vi "Encoder SD Write.vi"(9 "Encoder Data":T1 {"Ticks" format="%#.6g"}, 11 "Name":string) -> ()   [LabVIEW 2013]
uses:
  Single Encoder Data.ctl
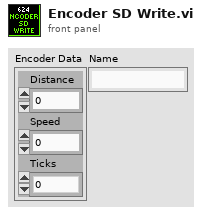
[diagram p1: front panel]
types:
  T1 = typedef "Single Encoder Data.ctl" = cluster{"Distance":dbl, "Speed":dbl, "Ticks":dbl}
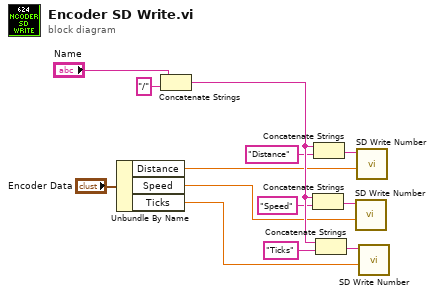
[diagram p0: block diagram]
diagram:
  n1 = Unbundle By Name("Encoder Data") -> ("Distance"=w3:dbl, "Speed"=w2:dbl, "Ticks"=w1:dbl)
  n2 = Concatenate Strings("Name", "/" ("string")) -> (w10:string)
  n3 = Concatenate Strings(w10, "Speed" ("string")) -> (w5:string)
  n4 = Concatenate Strings(w10, "Distance" ("string")) -> (w4:string)
  n5 = Concatenate Strings(w10, "Ticks" ("string")) -> (w6:string)
  n6 = call <vilib>:"SD Write Number.vi"("Numeric"=w2, "Name"=w5) -> ()  [unwired: 8 in, 2 out]
  n7 = call <vilib>:"SD Write Number.vi"("Numeric"=w3, "Name"=w4) -> ()  [unwired: 8 in, 2 out]
  n8 = call <vilib>:"SD Write Number.vi"("Numeric"=w1, "Name"=w6) -> ()  [unwired: 8 in, 2 out]
